vi "QPosition.vi"(8 "error in (no error)":errorcluster, 10 "Axis":i32=1, 11 "VISA resource name in":refnum<visa-resource-name>) -> (0 "error out":errorcluster, 2 "Position":dbl, 3 "VISA resource name out":refnum<visa-resource-name>)   [LabVIEW 2015]
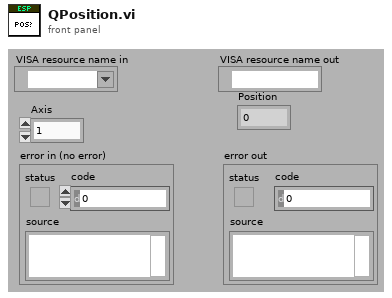
[diagram p1: front panel]
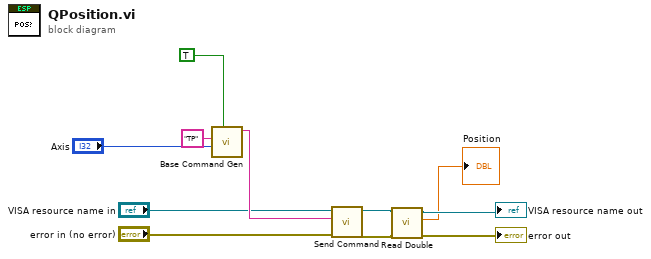
[diagram p0: block diagram]
diagram:
  n1 = call "Base Command Gen.vi"("Query"=TRUE, "Command"="TP", "xx"="Axis") -> ("Command"=w10:string)  [unwired: 8 in]
  n2 = call "Send Command.vi"("error out (no error)"="error in (no error)", "Command"=w10, "VISA resource name in"="VISA resource name in") -> ("error out"=w4:errorcluster, "VISA resource name out"=w5:refnum<visa-resource-name>)  [unwired: 7 in]
  n3 = call "Read Double.vi"("error in (no error)"=w4, "VISA resource name"=w5) -> ("error out"=→"error out":errorcluster, "Double"=→"Position":dbl, "VISA resource name out"=→"VISA resource name out":refnum<visa-resource-name>)  [unwired: 7 in]
